vi "Digital Multiple.vi"(8 "error in (no error)":errorcluster, 9 "Data":T1, 11 "ValveControlModule in":refnum<class "ValveControlModule.lvclass">) -> (0 "error out":errorcluster, 3 "ValveControlModule out":refnum<class "ValveControlModule.lvclass">)   [LabVIEW 2020, in "VolatusControl.lvlib" / "ValveControlModule.lvclass"]
uses:
  ValveControlModule.lvclass
  ValveControlModule.lvclass/ValveControlModule.ctl
  Valve/ValveControl.lvclass
  messages/CmdDigital/Data.ctl
  messages/CmdDigital/CmdDigital.lvlib
  messages/CmdDigitalMultiple/Data.ctl
  messages/CmdDigitalMultiple/CmdDigitalMultiple.lvlib
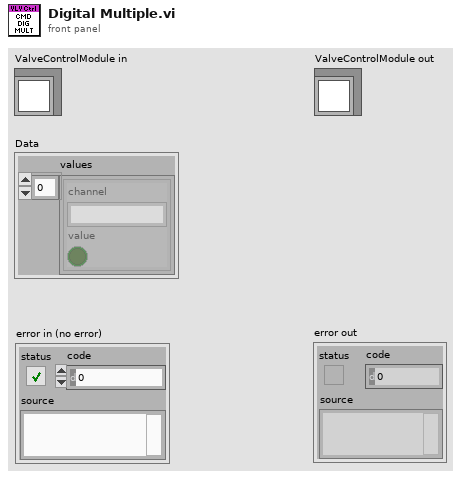
[diagram p1: front panel]
types:
  T1 = typedef "CmdDigitalMultiple.lvlib/Data.ctl" = cluster{"values":T2[]}
  T2 = typedef "CmdDigital.lvlib/Data.ctl" = cluster{"channel":string, "value":bool}
  T3 = map{string, refnum<class "ValveControl.lvclass">}
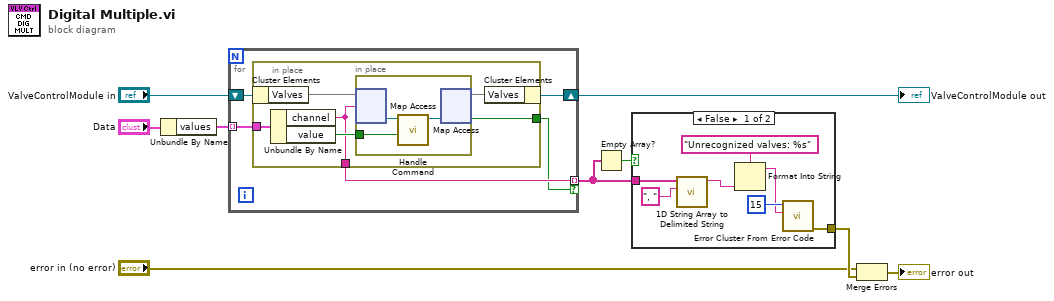
[diagram p0: block diagram]
diagram:
  n1 = Unbundle By Name("Data") -> ("values"=w9:T2[])
  n2 = for {
    shift-right: [w13] -> w4
    shift-left: "ValveControlModule in" -> [w14]
    tunnel: w9 -> [w12] mode=indexing
    tunnel: [w11] -> w7 mode=indexing if=w10
    n3 = in-place {
      in-place-border: [w17] -> w10
      in-place-border: [w15] -> w11
      in-place-border: w12 -> [w16]
      n4 = in-place-cluster #1(w14) -> ("Valves"=w20:T3)
      n5 = Unbundle By Name(w16) -> ("channel"=w15:string, "value"=w19:bool)
      n6 = in-place {
        in-place-border: w19 -> [w21]
        n7 = in-place-map #2(w20, w15) -> (w23:refnum<class "ValveControl.lvclass">)  [unwired: 1 in, 1 out]
        n8 = call-dynamic "Handle Command.vi"("Value"=w21, "Valve in"=w23) -> ("Valve out"=w22:refnum<class "ValveControl.lvclass">)  [unwired: 8 in, 1 out]
        n9 = in-place-map #2(w22) -> (w18:T3, w17:bool)  [unwired: 1 in, 1 out]
      }
      n10 = in-place-cluster #1("Valves"=w18) -> (w13:refnum<class "ValveControlModule.lvclass">)
    }
  }
  "ValveControlModule out" <- w4
  n11 = Empty Array?(array=w7) -> (empty?=w8:bool)
  n12 = case shown="False" w8 {
    tunnel: [w27 _] -> w3
    tunnel: w7 -> [w26 _]
    frame False {
      n13 = call <vilib>:"1D String Array to Delimited String.vi"("delimiter"=", ", "string array"=w26) -> ("delimited string"=w24:string)  [unwired: 9 in]
      n14 = Format Into String(format string="Unrecognized valves: %s", w24) -> (resulting string=w28:string)  [unwired: 2 in, 1 out]
      n15 = call <vilib>:"Error Cluster From Error Code.vi"("error message (\"\")"=w28, "error code (0)"=15) -> ("error out"=w27:errorcluster)  [unwired: 7 in]
    }
    frame True {
    }
  }
  n16 = Merge Errors("error in (no error)", w3) -> (→"error out":errorcluster)
